vi "fullPath.vi"(1 "file path (dialog if empty)":path) -> (0 "full path":path)   [LabVIEW 2021]
uses:
  <vilib>/Utility/file.llb/Write Delimited Spreadsheet (string).vi
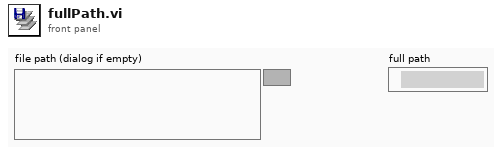
[diagram p1: front panel]
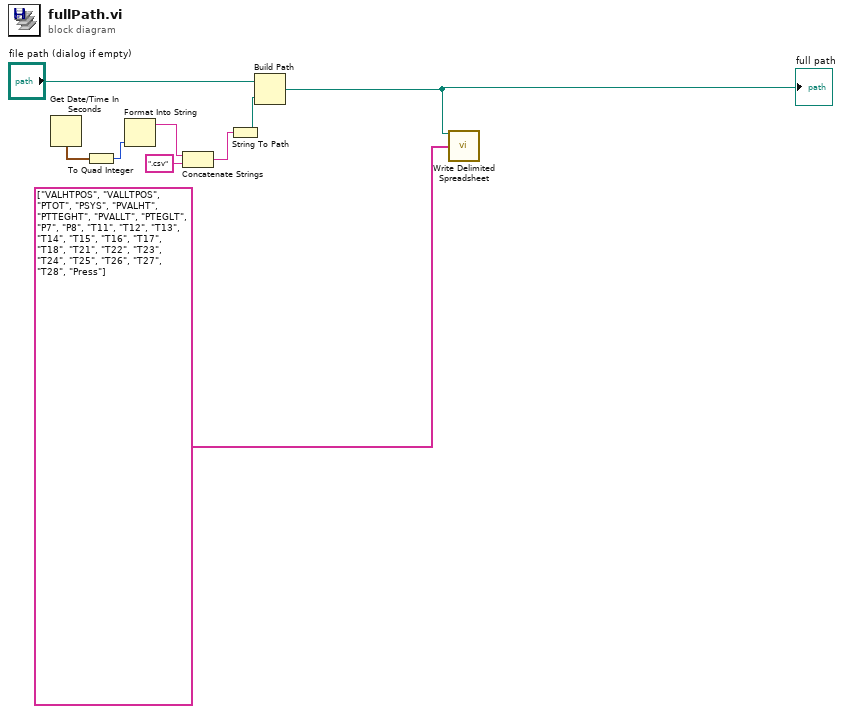
[diagram p0: block diagram]
diagram:
  n1 = Get Date/Time In Seconds() -> (seconds since 1Jan1904=w5:timestamp)
  n2 = To Quad Integer(1:w5) -> (0:w4:i64)
  n3 = Format Into String(w4) -> (resulting string=w3:string)  [unwired: 3 in, 1 out]
  n4 = Concatenate Strings(w3, ".csv" ("string")) -> (w1:string)
  n5 = String To Path(string=w1) -> (path=w7:path)
  n6 = Build Path(base path="file path (dialog if empty)", name or relative path=w7) -> (appended path=w6:path)
  "full path" <- w6
  n7 = call-poly <vilib>:"Write Delimited Spreadsheet.vi"("file path (dialog if empty)"=w6, "1D data"=string[] ["VALHTPOS", "VALLTPOS", "PTOT", "PSYS", "PVALHT", "PTTEGHT", "PVALLT", "PTEGLT", "P7", "P8", "T11", "T12", "T13", "T14", "T15", "T16", "T17", "T18", "T21", "T22", "T23", "T24", "T25", "T26", "T27", "T28", "Press"] ("Array")) -> ()  [unwired: 12 in, 2 out]
